vi "strings to line.vi"(11 "strings":string[](array[string])) -> (3 "line":T1)   [LabVIEW 2013, in "EIP Tags editor node.lvclass"]
uses:
  EIP Tags editor node.lvclass
  table line.ctl
  channel/EIP Tags Channel.lvclass
  <vilib>/NI/Tag Bus Module Framework/channel/channel classification.ctl
  <vilib>/NI/Tag Bus Module Framework/channel/TBM channel.lvclass
  configuration/EIP Tags Configuration.lvclass
  configuration/eip tag types.ctl
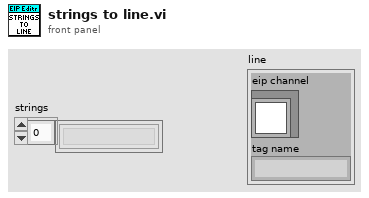
[diagram p1: front panel]
types:
  T1 = typedef "EIP Tags editor node.lvclass/table line.ctl" = cluster{"eip channel":refnum<class "EIP Tags Channel.lvclass">, "tag name":string}
  T2 = typedef "EIP Tags Configuration.lvclass/eip tag types.ctl" = enum16{"SINT", "INT", "DINT", "REAL", "BOOL", "STRING"}
  T3 = typedef "TBM channel.lvclass/channel classification.ctl" = enum16{"input data", "output data", "processing parameter", "processing result"}
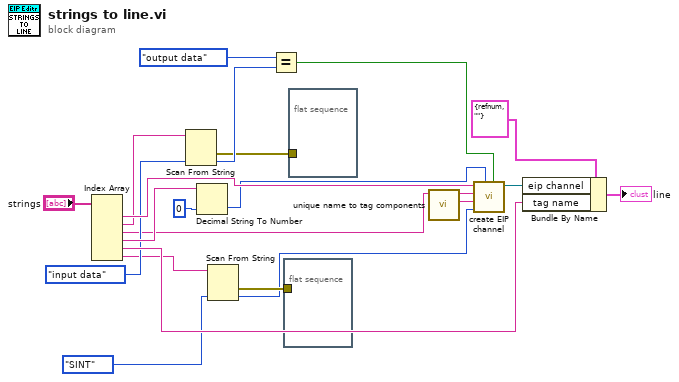
[diagram p0: block diagram]
diagram:
  n1 = Index Array(array="strings") -> (element #1=w18:string, element #2=w13:string, element #3=w5:string, element #4=w15:string, element #5=w19:string, element #6=w1:string)  [unwired: 6 in]
  n2 = Scan From String(input string=w13, default 1=channel_classification."input data" ("channel classification")) -> (error out=w8:errorcluster, output 1=w11:T3)  [unwired: 3 in, 2 out]
  n3 = Decimal String To Number(string=w15, default (0L)=u32 0 ("default (0 I32)")) -> (number=w14:u32)  [unwired: 1 in, 1 out]
  n4 = Scan From String(input string=w1, default 1=eip_tag_types."SINT" ("eip tag type")) -> (error out=w4:errorcluster, output 1=w3:T2)  [unwired: 3 in, 2 out]
  n5 = Equal?(x=channel_classification."output data", y=w11) -> (x = y?=w9:bool)
  n6 = flat-sequence {
    tunnel: w4 -> [_]
    frame #0 {
    }
  }
  n7 = flat-sequence {
    tunnel: w8 -> [_]
    frame #0 {
    }
  }
  n8 = call "unique name to tag components.vi"("unique name"=w5) -> ("Tag Name"=w6:string, "Network Path"=w7:string)  [unwired: 9 in]
  n9 = call "create EIP channel.vi"("output?"=w9, "element index"=w14, "eip tag type"=w3, "Tag Name"=w6, "Network Path"=w7, "name"=w18) -> ("EthernetIP Channel out"=w17:refnum<class "EIP Tags Channel.lvclass">)  [unwired: 5 in]
  n10 = Bundle By Name(cluster=T1 {"eip channel"=refnum, "tag name"=""} ("line"), "eip channel"=w17, "tag name"=w19) -> (→"line":T1)
